vi "_CallDirectly.vi"() -> ()   [LabVIEW 2019, in "lv-classprovidershell-example.lvlib"]
uses:
  lv-classprovidershell-example.lvlib
  content/ContentClass1/ContentClass1.lvclass
panel:
  out "valid":bool
  # "[Example] Call content class directly\n\nRun this VI."
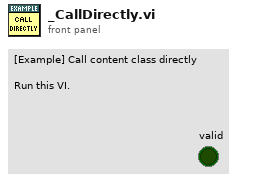
[diagram p1: front panel]
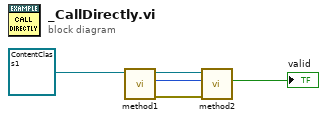
[diagram p0: block diagram]
diagram:
  n1 = call-dynamic "method1.vi"("ContentClass in"=refnum<class "ContentClass1.lvclass"> refnum ("lv-providershell-example3.lvlib:ContentClass.lvclass")) -> ("error out"=w3:errorcluster, "RefNum"=w4:i32, "ContentClass out"=w5:refnum<class "ContentClass1.lvclass">)  [unwired: 8 in]
  n2 = call-dynamic "method2.vi"("error in (no error)"=w3, "RefNum"=w4, "ContentClass in"=w5) -> ("Boolean"=→"valid":bool)  [unwired: 6 in, 2 out]
